vi "PH_Beckhoff_PP_PU.get RR Tagname.vi"(1 "Ross Relais Tag":T2, 2 "PU":T1) -> (0 "RR Tagname":string)   [LabVIEW 2014, in "PH_Beckhoff_PP_PU.lvlib"]
doc: "This VI concatenates a Tagname out of strict type def enum controls. It keeps also the information whether the Tag is existing (if not, N/A is given out as name)."
uses:
  PH_Beckhoff_PP_PU.lvlib
  PH_Beckhoff_PP_PU.RR Tags.ctl
  PH_Basics/PH_PP_Common/PH_PP_Common.PUs.ctl
  PH_Basics/PH_Common/Names/PH_Names.Subsystems.ctl
  PH_Basics/PH_PP_Common/PH_PP_Common.Devices.ctl
  PH_Basics/PH_Common/Names/PH_Names.Communication Type.ctl
  PH_Basics/PH_Common/PH_Common.lvlib
  PH_Basics/PH_PP_Common/PH_PP_Common.lvlib
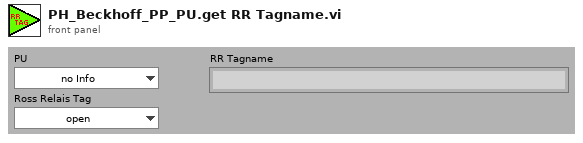
[diagram p1: front panel]
types:
  T1 = typedef "PH_PP_Common.lvlib/PH_PP_Common.PUs.ctl" = enum16{"no Info", "PA-19mm-1", "PA-19mm-2", "PA-45mm-PILC", "PA-45mm-MAIN", "MA-PU-1", "MA-PU-2", "MA-PU-3", "MA-PU-4", "MA-PU-5", "MA-PU-6", "MA-FR", "MA-PILC", "PA-45mm-DP"}
  T2 = typedef "PH_Beckhoff_PP_PU.lvlib/PH_Beckhoff_PP_PU.RR Tags.ctl" = enum16{"open", "closed", "close", "Status"}
  T3 = typedef "PH_Common.lvlib/PH_Names.Subsystems.ctl" = enum16{"no Info", "fs-FE", "ns-FE", "PA", "MA", "MAS", "COS", "Exp-LB", "Exp-LL", "PP", "PILS"}
  T4 = typedef "PH_PP_Common.lvlib/PH_PP_Common.Devices.ctl" = enum16{"no Info", "Igni", "RR", "DumpRoss", "PSU", "Trigger", "HV-Meas", "Rods", "Chiller", "Conductivity", "Mercury"}
  T5 = typedef "PH_Common.lvlib/PH_Names.Communication Type.ctl" = enum16{"no Info", "SE", "SA", "AE", "AA", "DE", "DA", "DIM"}
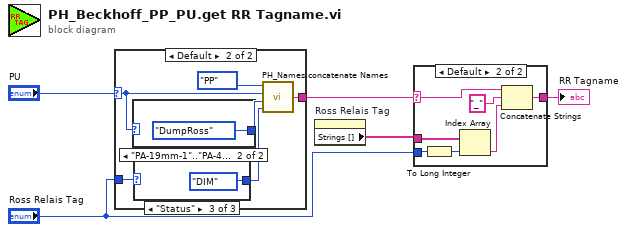
[diagram p0: block diagram]
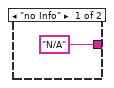
[diagram p2: hidden frame]
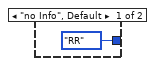
[diagram p3: hidden frame]
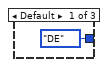
[diagram p4: hidden frame]
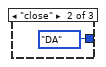
[diagram p5: hidden frame]
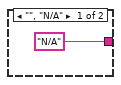
[diagram p6: hidden frame]
diagram:
  n1 = case shown="Default" "PU" {
    selector: "PU" -> [_ w7]
    tunnel: ["N/A" ("Subsystem_PU_Devices_Comm Type") w12] -> w4
    tunnel: "Ross Relais Tag" -> [_ w11]
    frame "no Info" {
    }
    frame Default {
      n2 = case shown="\"PA-19mm-1\"..\"PA-45mm-MAIN\"" w7 {
        tunnel: [PH_PP_Common.Devices."RR" ("Devices (no info)") PH_PP_Common.Devices."DumpRoss" ("Devices (no info)")] -> w10
        frame "no Info", Default {
        }
        frame "PA-19mm-1".."PA-45mm-MAIN" {
        }
      }
      n3 = case shown="\"Status\"" w11 {
        tunnel: [PH_Names.Communication_Type."DE" ("Communication Type (no info)") PH_Names.Communication_Type."DA" ("Communication Type (no info)") PH_Names.Communication_Type."DIM" ("Communication Type (no info)")] -> w8
        frame Default {
        }
        frame "close" {
        }
        frame "Status" {
        }
      }
      n4 = call "PH_Names.concatenate Names.vi"("Communication Type (no info)"=w8, "Devices (no info)"=w10, "PU (no info)"=w7, "Subsystem"=PH_Names.Subsystems."PP") -> ("Subsystem_PU_Devices_Comm Type"=w12:string)
    }
  }
  n5 = property on="Ross Relais Tag" class="Enum (strict)"() -> ("Strings []"=w3:string[])  [unwired: 2 in, 2 out]
  n6 = case shown="Default" w4 {
    selector: w4 -> [_ w19]
    tunnel: ["N/A" w25] -> w5
    tunnel: w3 -> [_ w24]
    tunnel: "Ross Relais Tag" -> [_ w20]
    frame "", "N/A" {
    }
    frame Default {
      n7 = To Long Integer(number=w20) -> (32bit integer=w23:i32)
      n8 = Index Array(array=w24, index=w23) -> (element=w22:string)
      n9 = Concatenate Strings(w19, "_" ("string"), w22) -> (w25:string)
    }
  }
  "RR Tagname" <- w5
